vi "HEWH Check Full Credit Draw.vi"(7 "Draw_Start":dbl, 8 "error in (no error)":errorcluster, 10 "Upper Most Element":T1=enum."Lower Element", 11 "UEF Calculated Values Input in":T2 {"Data Indexes"."15 sec after Draw Index" format="%#.2f"; "Data Indexes"."15 sec after Draw Timestamp" format="%#.2f"; "Data Indexes"."Test Start Timestamp" format="%.2f"; "Data Indexes"."Test End Timestamp" format="%.2f"; "Data Indexes"."T0 Timestamp" format="%.2f"; "Data Indexes"."Tsf Timestamp" format="%.2f"; "Data Indexes"."Tsu0 Timestamp" format="%.2f"; "Data Indexes"."Tmax1 Timestamp" format="%.2f"; "Data Indexes"."Draw Index Timestamp" format="%#.2f"; "Data Indexes"."Non-Draw Timestamp" format="%#.2f"; "Data Indexes"."Heating Timestamp" format="%#.2f"; "Data Indexes"."Start Energy (BTU-Gas)" format="%.6f"; "Data Indexes"."Start Watt Hours" format="%.6f"; "Static Data"."V - Volume of Wh (True)" format="%.5f"; "Static Data"."T-Ambinet Nominal (°F)" format="%.5f"; "Static Data"."T-Inlet Setpoint (°F)" format="%.5f"; "Static Data"."T-Wh Setpoint (°F)" format="%.5f"; "Sampled Data"."Qe (Wh)" format="%.5f"; "Sampled Data"."Tau stby2 (hr)" format="%.5f"; "Sampled Data"."Tastby2 (°F)" format="%.5f"; "Sampled Data"."Qf (BTU)" format="%.5f"; "Sampled Data"."Qe (BTU)" format="%.5f"; "Sampled Data"."Tmax1 (°F)" format="%.5f"; "Sampled Data"."T0 (°F)" format="%.5f"; "Sampled Data"."Qr (BTU)" format="%.5f"; "Sampled Data"."T 24(°F)" format="%.5f"; "Sampled Data"."T astby(°F)" format="%.5f"; "Sampled Data"."T tstby(°F)" format="%.5f"; "Sampled Data"."T su0(°F)" format="%.5f"; "Sampled Data"."T suf(°F)" format="%.5f"; "Sampled Data"."Tau stby_1 (hr)" format="%.5f"; "Sampled Data"."Qsuf (BTU)" format="%.5f"; "Sampled Data"."Qsu0 (BTU)" format="%.5f"; "Calculated Values"."Draw Bonus Volume (gal)" format="%.6f"; "Calculated Values"."Adjustment Factor" format="%.6f"; "Calculated Values"."T*avg_del(n-1)" format="%.6f"; "Calculated Values"."T*min(n-1)" format="%.6f"; "Calculated Values"."T*avg_del(n)" format="%.6f"; "Calculated Values"."Vn" format="%.6f"; "Calculated Values"."Qdm (BTU)" format="%.6f"; "Calculated Values"."QHWD (BTU)" format="%.6f"; "Calculated Values"."QHW (BTU)" format="%.6f"; "Calculated Values"."UEF" format="%.6f"; "Calculated Values"."QHW67 (BTU)" format="%.6f"; "Calculated Values"."Qda (BTU)" format="%.6f"; "Calculated Values"."Qd (BTU)" format="%.6f"; "Calculated Values"."Q (BTU)" format="%.6f"; "Calculated Values"."UA (BTU/(hr*F))" format="%.6f"; "Calculated Values"."Qhr (BTU/hr)" format="%.6f"; "Calculated Values"."Qstby (BTU)" format="%.6f"; "Calculated Values"."nu_r" format="%.6f"; "Calculated Values"."CpUEF (BTU/(lb*F))" format="%.6f"; "Calculated Values"."rho_nu (lb/gal)" format="%.6f"; "Calculated Values"."V1- Vol (Gal)" format="%.6f"; "Calculated Values"."M cluster mass removed (lb)" format="%.6f"; "Calculated Values"."Cp theoretical (BTU/(lbm °F))" format="%.6f"; "Calculated Values"."Tin1 - Mean Inlet 1st Cluster (°F)" format="%.6f"; "Calculated Values"."Tdel1-Mean Outlet 1st Cluster(°F)" format="%.6f"; "Calculated Values"."Cp 24 (BTU/(lb*F))" format="%.6f"; "Calculated Values"."Cp standby (BTU/(lb*F))" format="%.6f"; "Calculated Values"."Cp2 (BTU/(lb*F))" format="%.6f"; "Calculated Values"."Cp1 (BTU/(lb*F))" format="%.6f"; "Calculated Values"."rho 24 (lb/gal)" format="%.6f"; "Calculated Values"."rho standby (lb/gal)" format="%.6f"; "Calculated Values"."rho 2 (lb/gal)" format="%.6f"; "Calculated Values"."Density of cold water All (lbm/gal)" format="%#.3g"; "Calculated Values"."CpHW (BTU/(lbm °F))" format="%#.3g"; "Calculated Values"."Density of hot water All (lbm/gal)" format="%#.3g"; "Calculated Values"."Mass of water All (lbm)" format="%#.3f"}) -> (0 "error out":errorcluster, 2 "Flow Type":T4, 3 "UEF Calculated Values Output":T2 {"Data Indexes"."15 sec after Draw Index" format="%#.2f"; "Data Indexes"."15 sec after Draw Timestamp" format="%#.2f"; "Data Indexes"."Test Start Timestamp" format="%.2f"; "Data Indexes"."Test End Timestamp" format="%.2f"; "Data Indexes"."T0 Timestamp" format="%.2f"; "Data Indexes"."Tsf Timestamp" format="%.2f"; "Data Indexes"."Tsu0 Timestamp" format="%.2f"; "Data Indexes"."Tmax1 Timestamp" format="%.2f"; "Data Indexes"."Draw Index Timestamp" format="%#.2f"; "Data Indexes"."Non-Draw Timestamp" format="%#.2f"; "Data Indexes"."Heating Timestamp" format="%#.2f"; "Data Indexes"."Start Energy (BTU-Gas)" format="%.6f"; "Data Indexes"."Start Watt Hours" format="%.6f"; "Static Data"."V - Volume of Wh (True)" format="%.5f"; "Static Data"."T-Ambinet Nominal (°F)" format="%.5f"; "Static Data"."T-Inlet Setpoint (°F)" format="%.5f"; "Static Data"."T-Wh Setpoint (°F)" format="%.5f"; "Sampled Data"."Qe (Wh)" format="%.5f"; "Sampled Data"."Tau stby2 (hr)" format="%.5f"; "Sampled Data"."Tastby2 (°F)" format="%.5f"; "Sampled Data"."Qf (BTU)" format="%.5f"; "Sampled Data"."Qe (BTU)" format="%.5f"; "Sampled Data"."Tmax1 (°F)" format="%.5f"; "Sampled Data"."T0 (°F)" format="%.5f"; "Sampled Data"."Qr (BTU)" format="%.5f"; "Sampled Data"."T 24(°F)" format="%.5f"; "Sampled Data"."T astby(°F)" format="%.5f"; "Sampled Data"."T tstby(°F)" format="%.5f"; "Sampled Data"."T su0(°F)" format="%.5f"; "Sampled Data"."T suf(°F)" format="%.5f"; "Sampled Data"."Tau stby_1 (hr)" format="%.5f"; "Sampled Data"."Qsuf (BTU)" format="%.5f"; "Sampled Data"."Qsu0 (BTU)" format="%.5f"; "Calculated Values"."Draw Bonus Volume (gal)" format="%.6f"; "Calculated Values"."Adjustment Factor" format="%.6f"; "Calculated Values"."T*avg_del(n-1)" format="%.6f"; "Calculated Values"."T*min(n-1)" format="%.6f"; "Calculated Values"."T*avg_del(n)" format="%.6f"; "Calculated Values"."Vn" format="%.6f"; "Calculated Values"."Qdm (BTU)" format="%.6f"; "Calculated Values"."QHWD (BTU)" format="%.6f"; "Calculated Values"."QHW (BTU)" format="%.6f"; "Calculated Values"."UEF" format="%.6f"; "Calculated Values"."QHW67 (BTU)" format="%.6f"; "Calculated Values"."Qda (BTU)" format="%.6f"; "Calculated Values"."Qd (BTU)" format="%.6f"; "Calculated Values"."Q (BTU)" format="%.6f"; "Calculated Values"."UA (BTU/(hr*F))" format="%.6f"; "Calculated Values"."Qhr (BTU/hr)" format="%.6f"; "Calculated Values"."Qstby (BTU)" format="%.6f"; "Calculated Values"."nu_r" format="%.6f"; "Calculated Values"."CpUEF (BTU/(lb*F))" format="%.6f"; "Calculated Values"."rho_nu (lb/gal)" format="%.6f"; "Calculated Values"."V1- Vol (Gal)" format="%.6f"; "Calculated Values"."M cluster mass removed (lb)" format="%.6f"; "Calculated Values"."Cp theoretical (BTU/(lbm °F))" format="%.6f"; "Calculated Values"."Tin1 - Mean Inlet 1st Cluster (°F)" format="%.6f"; "Calculated Values"."Tdel1-Mean Outlet 1st Cluster(°F)" format="%.6f"; "Calculated Values"."Cp 24 (BTU/(lb*F))" format="%.6f"; "Calculated Values"."Cp standby (BTU/(lb*F))" format="%.6f"; "Calculated Values"."Cp2 (BTU/(lb*F))" format="%.6f"; "Calculated Values"."Cp1 (BTU/(lb*F))" format="%.6f"; "Calculated Values"."rho 24 (lb/gal)" format="%.6f"; "Calculated Values"."rho standby (lb/gal)" format="%.6f"; "Calculated Values"."rho 2 (lb/gal)" format="%.6f"; "Calculated Values"."Density of cold water All (lbm/gal)" format="%#.3g"; "Calculated Values"."CpHW (BTU/(lbm °F))" format="%#.3g"; "Calculated Values"."Density of hot water All (lbm/gal)" format="%#.3g"; "Calculated Values"."Mass of water All (lbm)" format="%#.3f"})   [LabVIEW 2023]
uses:
  Type Definitions/HEWH FHR Draw Type.ctl
  Type Definitions/UEF Constants.ctl
  Type Definitions/HEWH Draw Stats.ctl
  Type Definitions/FHR Bins.ctl
  Type Definitions/HEWH Meter Type.ctl
  Type Definitions/Upper Most Element.ctl
panel:
  out "Time Heating Turned Off":dbl
  # "FHR"
  # "FHR"
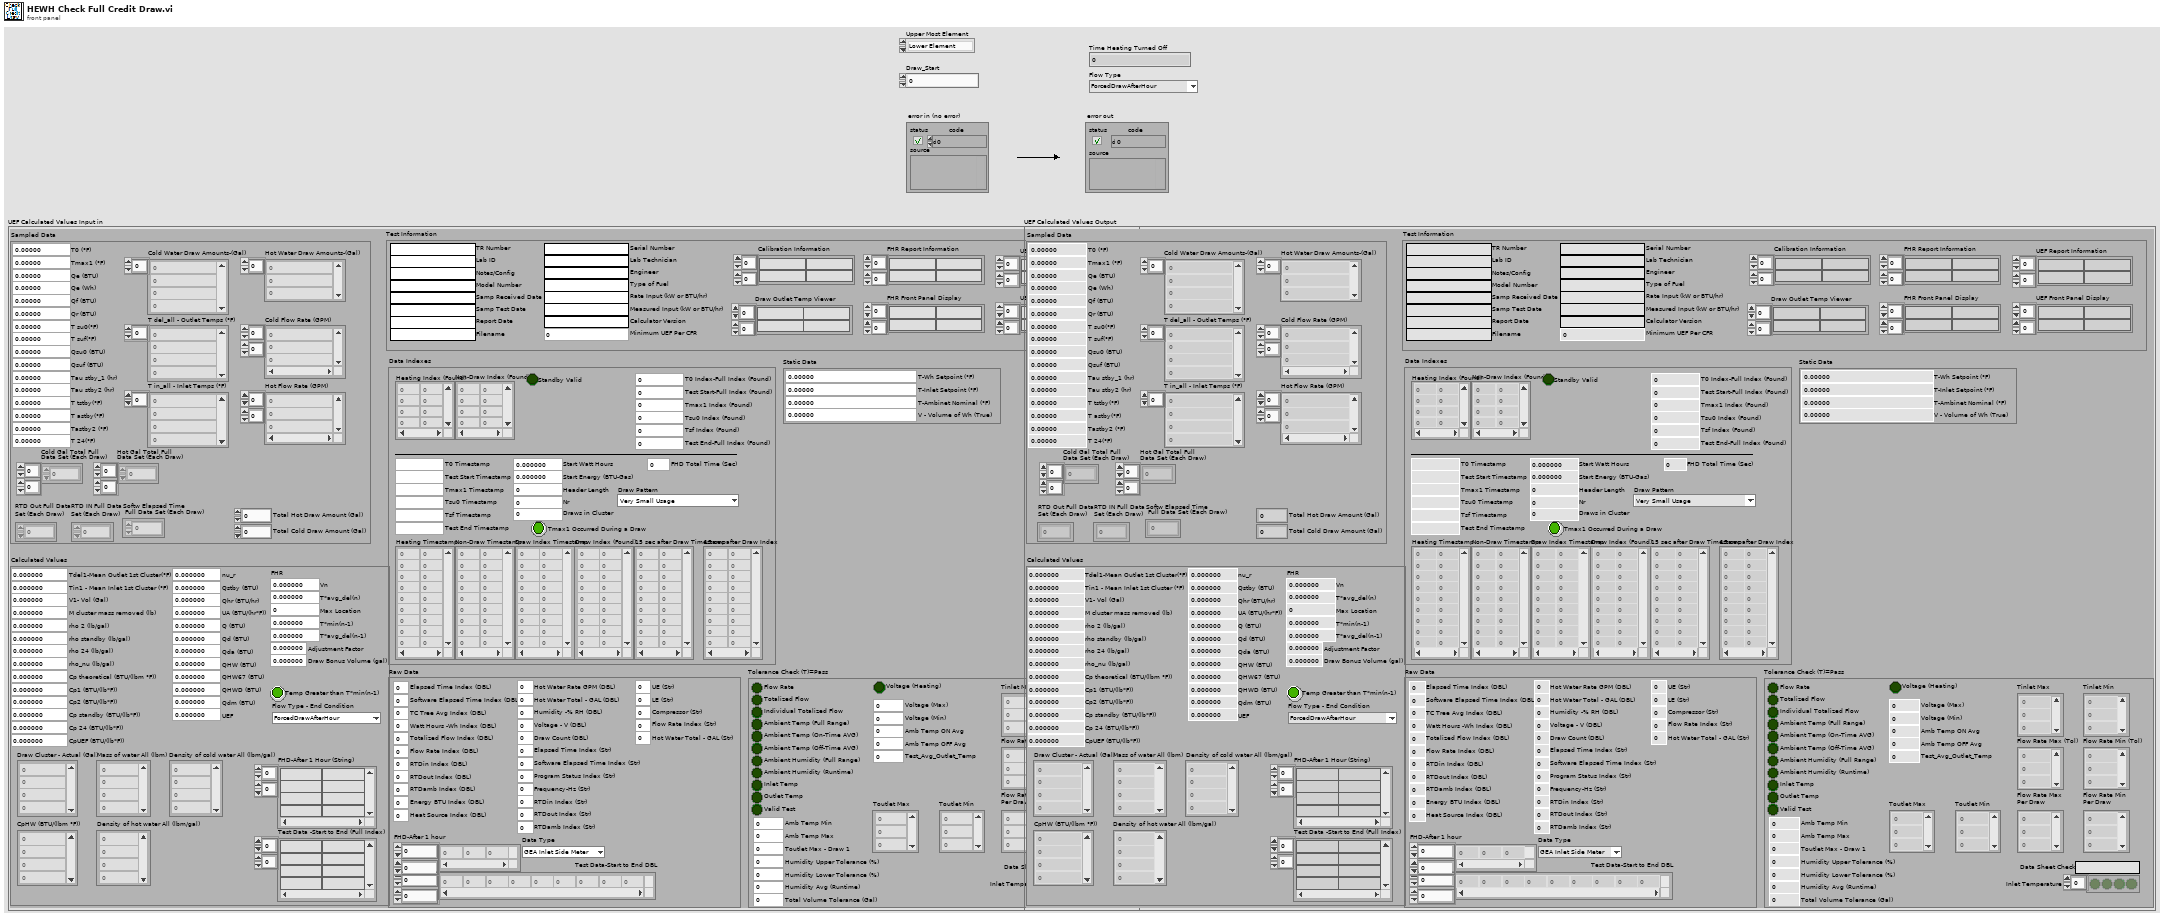
[diagram p1: front panel]
types:
  T1 = typedef "Upper Most Element.ctl" = enum16{"Compressor", "Lower Element", "Upper Element"}
  T2 = typedef "UEF Constants.ctl" = cluster{"Calculated Values":T3, "Sampled Data":cluster{"Cold Water Draw Amounts-(Gal)":dbl[], "T del_all - Outlet Temps (°F)":dbl[], "T in_all - Inlet Temps (°F)":dbl[], "Qsu0 (BTU)":dbl, "Qsuf (BTU)":dbl, "Tau stby_1 (hr)":dbl, "T suf(°F)":dbl, "T su0(°F)":dbl, "T tstby(°F)":dbl, "T astby(°F)":dbl, "T 24(°F)":dbl, "Qr (BTU)":dbl, "T0 (°F)":dbl, "Tmax1 (°F)":dbl, "Qe (BTU)":dbl, "Qf (BTU)":dbl, "Tastby2 (°F)":dbl, "RTD Out Full Data\nSet (Each Draw)":dbl[][], "RTD IN Full Data\nSet (Each Draw)":dbl[][], "Tau stby2 (hr)":dbl, "Hot Water Draw Amounts-(Gal)":dbl[], "Cold Flow Rate (GPM)":dbl[][], "Hot Flow Rate (GPM)":dbl[][], "Softw Elapsed Time\n Full Data Set (Each Draw)":dbl[][], "Cold Gal Total Full\nData Set (Each Draw)":dbl[][], "Total Hot Draw Amount (Gal) ":dbl, "Total Cold Draw Amount (Gal)":dbl, "Qe (Wh)":dbl, "Hot Gal Total Full\nData Set (Each Draw)":dbl[][]}, "Static Data":cluster{"T-Wh Setpoint (°F)":dbl, "T-Inlet Setpoint (°F)":dbl, "T-Ambinet Nominal (°F)":dbl, "V - Volume of Wh (True)":dbl}, "Data Indexes":cluster{"Test Start-Full Index (Found)":i32, "Header Length":i32, "Draw Index (Found)":i32[][], "Nr":i32, "Start Watt Hours":dbl, "Tsu0 Index (Found)":i32, "Tsf Index (Found)":i32, "Start Energy (BTU-Gas)":dbl, "Draws in Cluster":i32, "T0 Index-Full Index (Found)":i32, "Non-Draw Index (Found)":i32[][], "Tmax1 Index (Found)":i32, "Test End-Full Index (Found)":i32, "Heating Index (Found)":i32[][], "Heating Timestamp":dbl[][], "Non-Draw Timestamp":dbl[][], "Draw Index Timestamp":dbl[][], "Tmax1 Timestamp":dbl, "Tsu0 Timestamp":dbl, "Tsf Timestamp":dbl, "T0 Timestamp":dbl, "Test End Timestamp":dbl, "Test Start Timestamp":dbl, "15 sec after Draw Timestamp":dbl[][], "15 sec after Draw Index":dbl[][], "Tmax1 Occurred During a Draw":bool, "FHD Total Time (Sec)":dbl, "Draw Pattern":T5, "Standby Valid":bool}, "Raw Data":cluster{"Elapsed Time Index (DBL)":i32, "Software Elapsed Time Index (DBL)":i32, "TC Tree Avg Index (DBL)":i32, "Watt Hours -Wh Index (DBL)":i32, "Energy BTU Index (DBL)":i32, "Totalized Flow Index (DBL)":i32, "Flow Rate Index (DBL)":i32, "Program Status Index (Str)":i32, "RTDin Index (DBL)":i32, "RTDout Index (DBL)":i32, "RTDamb Index (DBL)":i32, "Test Data-Start to End DBL":dbl[][], "Data Type":T6, "Heat Source Index (DBL)":i32, "Hot Water Rate GPM (DBL)":i32, "Hot Water Total - GAL (DBL)":i32, "FHD-After 1 hour":dbl[][], "Humidity -% RH (DBL)":i32, "Voltage - V (DBL)":i32, "Draw Count (DBL)":i32, "Elapsed Time Index (Str)":i32, "Software Elapsed Time Index (Str)":i32, "Frequency-Hz (Str)":i32, "RTDin Index (Str)":i32, "RTDout Index (Str)":i32, "RTDamb Index (Str)":i32, "UE (Str)":i32, "LE (Str)":i32, "Compressor (Str)":i32, "Flow Rate Index (Str)":i32, "Hot Water Total - GAL (Str)":i32}, "Tolerance Check (T)=Pass":cluster{"Flow Rate":bool, "Totalized Flow":bool, "Ambient Temp (Full Range)":bool, "Ambient Humidity (Full Range)":bool, "Inlet Temp":bool, "Outlet Temp":bool, "Valid Test":bool, "Individual Totalized Flow":bool, "Data Sheet Check":string, "Inlet Temperature":bool[], "Tinlet Max":dbl[], "Tinlet Min":dbl[], "Flow Rate Max (Tol)":dbl[], "Flow Rate Min (Tol)":dbl[], "Amb Temp Max":dbl, "Amb Temp Min":dbl, "Toutlet Max - Draw 1":dbl, "Humidity Upper Tolerance (%)":dbl, "Total Volume Tolerance (Gal)":dbl, "Humidity Lower Tolerance (%)":dbl, "Flow Rate Max\nPer Draw":dbl[], "Flow Rate Min\nPer Draw":dbl[], "Ambient Humidity (Runtime)":bool, "Humidity Avg (Runtime)":dbl, "Ambient Temp (On-Time AVG)":bool, "Ambient Temp (Off-Time AVG)":bool, "Amb Temp OFF Avg":dbl, "Amb Temp ON Avg":dbl, "Voltage (Heating)":bool, "Voltage (Min)":dbl, "Voltage (Max)":dbl, "Toutlet Max":dbl[], "Toutlet Min":dbl[], "Test_Avg_Outlet_Temp":dbl}, "Test Information":cluster{"TR Number":string, "Lab ID":string, "Notes/Config":string, "Model Number":string, "Serial Number":string, "Lab Technician":string, "Engineer":string, "Type of Fuel":string, "Samp Received Date":string, "Samp Test Date":string, "Report Date":string, "Rate Input (kW or BTU/hr)":string, "Measured Input (kW or BTU/hr)":string, "Filename":string, "Calibration Information":string[][], "Calculator Version":string, "Minimum UEF Per CFR":dbl, "UEF Report Information":string[][], "FHR Report Information":string[][], "FHR Front Panel Display":string[][], "UEF Front Panel Display":string[][], "Draw Outlet Temp Viewer":string[][]}}
  T3 = typedef "HEWH Draw Stats.ctl" = cluster{"Draw Cluster - Actual (Gal)":dbl[], "Mass of water All (lbm)":dbl[], "Density of hot water All (lbm/gal)":dbl[], "CpHW (BTU/(lbm °F))":dbl[], "rho 2 (lb/gal)":dbl, "rho standby (lb/gal)":dbl, "rho 24 (lb/gal)":dbl, "Cp1 (BTU/(lb*F))":dbl, "Cp2 (BTU/(lb*F))":dbl, "Cp standby (BTU/(lb*F))":dbl, "Cp 24 (BTU/(lb*F))":dbl, "nu_r":dbl, "Qstby (BTU)":dbl, "Qhr (BTU/hr)":dbl, "UA (BTU/(hr*F))":dbl, "Q (BTU)":dbl, "Qd (BTU)":dbl, "Qda (BTU)":dbl, "QHW67 (BTU)":dbl, "UEF":dbl, "Tdel1-Mean Outlet 1st Cluster(°F)":dbl, "Tin1 - Mean Inlet 1st Cluster (°F)":dbl, "Cp theoretical (BTU/(lbm °F))":dbl, "M cluster mass removed (lb)":dbl, "V1- Vol (Gal)":dbl, "Test Data -Start to End (Full Index)":string[][], "rho_nu (lb/gal)":dbl, "Density of cold water All (lbm/gal)":dbl[], "CpUEF (BTU/(lb*F))":dbl, "QHW (BTU)":dbl, "QHWD (BTU)":dbl, "Qdm (BTU)":dbl, "FHD-After 1 Hour (String)":string[][], "Vn":dbl, "T*avg_del(n)":dbl, "Max Location":i32, "T*min(n-1)":dbl, "T*avg_del(n-1)":dbl, "Temp Greater than T*min(n-1)":bool, "Adjustment Factor":dbl, "Draw Bonus Volume (gal)":dbl, "Flow Type - End Condition":T4}
  T4 = typedef "HEWH FHR Draw Type.ctl" = enum16{"ForcedDrawAfterHour", "HeatingCutoffBeforeHour"}
  T5 = typedef "FHR Bins.ctl" = enum16{"Very Small Usage", "Low Usage", "Medium Usage", "High Usage", "Undefined"}
  T6 = typedef "HEWH Meter Type.ctl" = enum16{"GEA Inlet Side Meter", "GEA Outlet Side Meter", "CSA Inlet Side Meter"}
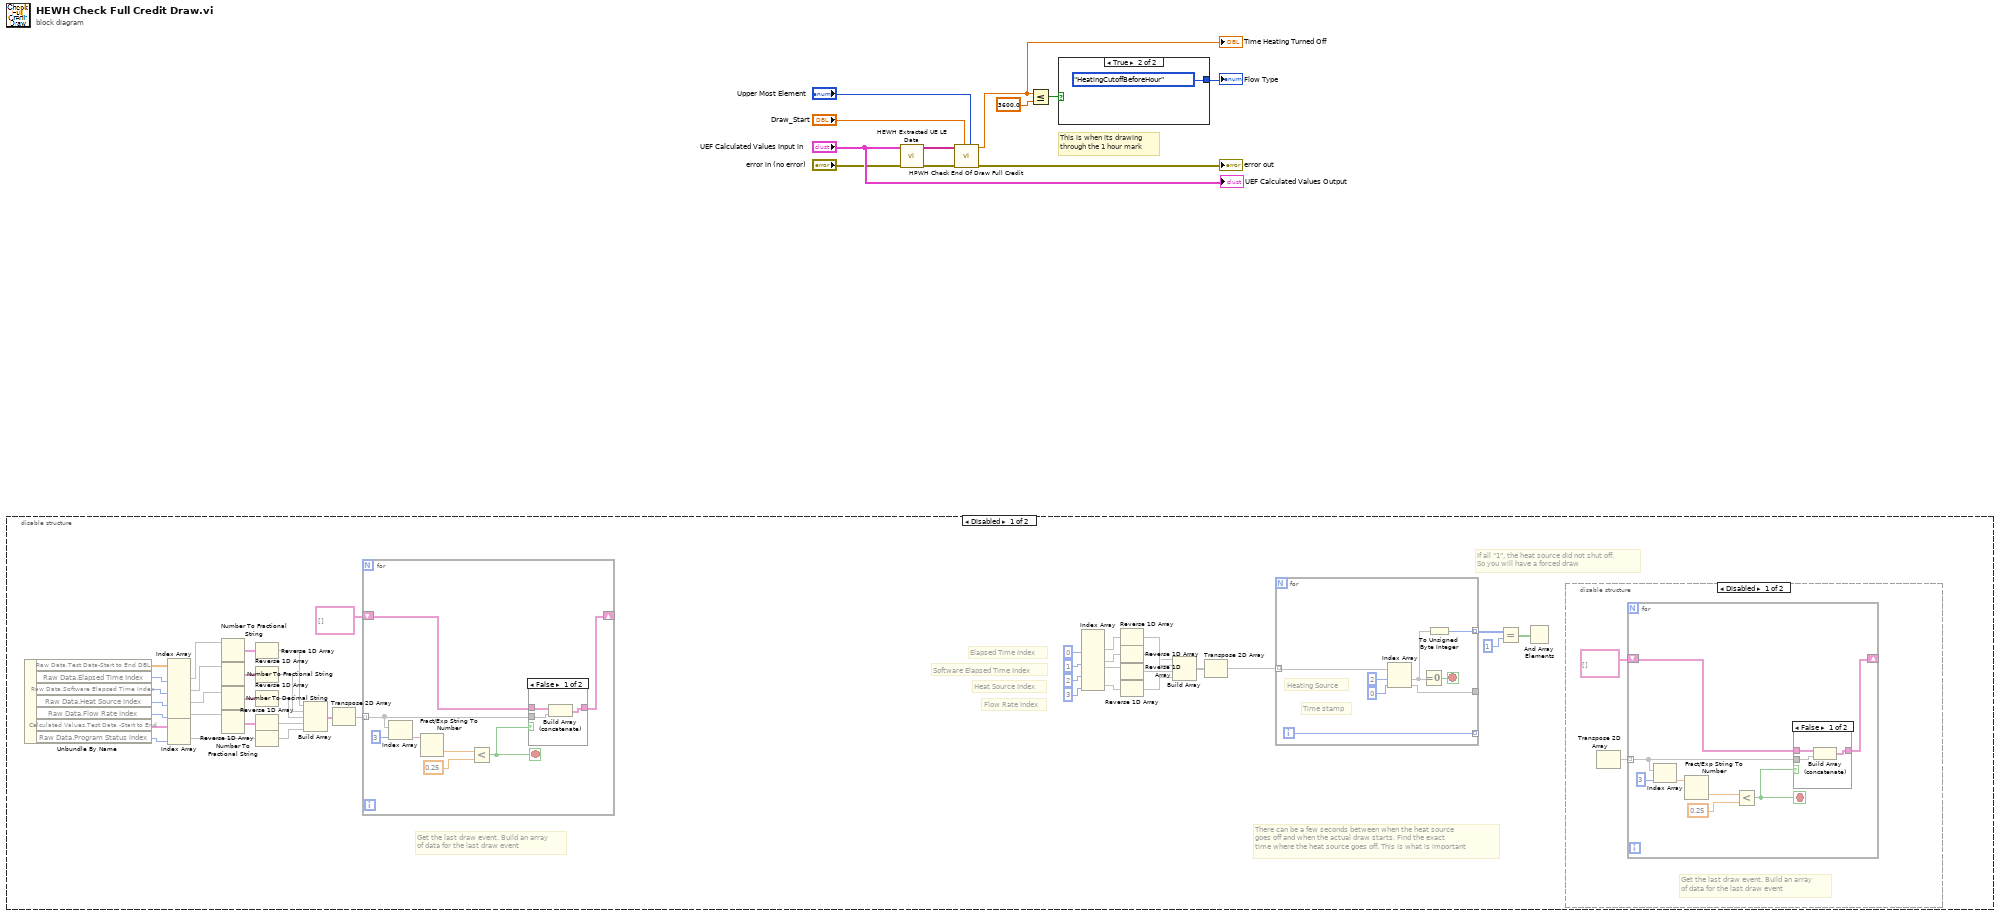
[diagram p0: block diagram]
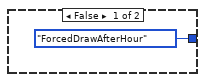
[diagram p2: hidden frame]
diagram:
  # "This is when its drawing\nthrough the 1 hour mark"
  n1 = disable-structure shown="Disabled" {
    frame Disabled {
      # "Get the last draw event. Build an array\nof data for the last draw event"
      # "If all \"1\", the heat source did not shut off.\nSo you will have a forced draw"
      # "Flow Rate Index"
      # "Heat Source Index"
      # "Software Elapsed Time Index"
      # "Elapsed Time Index"
      # "There can be a few seconds between when the heat source\ngoes off and when the actual draw starts. Find the exact\ntime where the heat source goes off. This is what is important"
      n2 = Unbundle By Name() -> ("Raw Data.Test Data-Start to End DBL"=w17:dbl[][], "Raw Data.Elapsed Time Index"=w16:i32, "Raw Data.Software Elapsed Time Index"=w15:i32, "Raw Data.Heat Source Index"=w14:i32, "Raw Data.Flow Rate Index"=w13:i32, "Calculated Values.Test Data -Start to End"=w24:string[][], "Raw Data.Program Status Index"=w25:i32)  [unwired: 1 in]
      n3 = Index Array(array=w17, index (col) #1=w16, index (col) #2=w15, index (col) #3=w14, index (col) #4=w13) -> (element #1=w27:dbl[], element #2=w29:dbl[], element #3=w31:dbl[], element #4=w33:dbl[])  [unwired: 4 in]
      n4 = Index Array(array=w24, index (col)=w25) -> (element=w26:string[])  [unwired: 1 in]
      n5 = Number To Fractional String(number=w27) -> (F-format string=w28:string[])  [unwired: 3 in]
      n6 = Number To Fractional String(number=w29) -> (F-format string=w30:string[])  [unwired: 3 in]
      n7 = Number To Decimal String(number=w31) -> (decimal integer string=w32:string[])  [unwired: 1 in]
      n8 = Number To Fractional String(number=w33) -> (F-format string=w34:string[])  [unwired: 3 in]
      n9 = Reverse 1D Array(array=w28) -> (reversed array=w21:string[])
      n10 = Reverse 1D Array(array=w30) -> (reversed array=w20:string[])
      n11 = Reverse 1D Array(array=w32) -> (reversed array=w19:string[])
      n12 = Reverse 1D Array(array=w34) -> (reversed array=w18:string[])
      n13 = Reverse 1D Array(array=w26) -> (reversed array=w23:string[])
      n14 = Build Array(w21, w20, w19, w18, w23) -> (w22:string[][])
      n15 = Transpose 2D Array(2D array=w22) -> (transposed array=w35:string[][])
      n16 = for {
        tunnel: w35 -> [w70] mode=indexing
        shift-right: [w71] -> _
        shift-left: string[][] [] -> [w72]
        stop <- w73 stop-if-true
        n17 = Index Array(array=w70, index=3) -> (element=w69:string)
        n18 = Fract/Exp String To Number(string=w69) -> (number=w67:dbl)  [unwired: 3 in, 1 out]
        n19 = Less?(x=w67, y=0.25) -> (x < y?=w73:bool)
        n20 = case shown="False" w73 {
          tunnel: [w76 w78] -> w71
          tunnel: w72 -> [w77 w78]
          tunnel: w70 -> [w75 _]
          frame False {
            n21 = Build Array (concatenate)(w77, w75) -> (w76:string[][])
          }
          frame True {
          }
        }
      }
      n22 = Index Array(index (col) #1=0 ("disabled index (col)"), index (col) #2=1 ("index (col)"), index (col) #3=2 ("index (col)"), index (col) #4=3 ("index (col)")) -> (element #1=w44, element #2=w45, element #3=w46, element #4=w47)  [unwired: 5 in]
      n23 = Reverse 1D Array(array=w44) -> (reversed array=w49:void[])
      n24 = Reverse 1D Array(array=w45) -> (reversed array=w50:void[])
      n25 = Reverse 1D Array(array=w46) -> (reversed array=w51:void[])
      n26 = Reverse 1D Array(array=w47) -> (reversed array=w52:void[])
      n27 = Build Array(w49, w50, w51, w52) -> (w48:void[])
      n28 = Transpose 2D Array(2D array=w48) -> (transposed array=w36:void[][])
      n29 = for {
        tunnel: w36 -> [w85] mode=indexing
        tunnel: [w82] -> _
        tunnel: [w81] -> _ mode=indexing
        tunnel: [w79] -> w39 mode=indexing
        i -> [w81]
        stop <- w84 stop-if-true
        # "Time stamp"
        # "Heating Source"
        n30 = Index Array(array=w85, index #1=2 ("index"), index #2=0 ("index")) -> (element #1=w80, element #2=w82)
        n31 = Equal To 0?(x=w80) -> (x = 0?=w84:bool)
        n32 = To Unsigned Byte Integer(number=w80) -> (unsigned 8bit integer=w79:u8)
      }
      n33 = Equal?(x=w39, y=u8 1) -> (x = y?=w37:bool[])
      n34 = And Array Elements(Boolean array=w37) -> ()  [unwired: 1 out]
      n35 = disable-structure shown="Disabled" {
        frame Disabled {
          # "Get the last draw event. Build an array\nof data for the last draw event"
          n36 = Transpose 2D Array() -> (transposed array=w53:dbl[][])  [unwired: 1 in]
          n37 = for {
            tunnel: w53 -> [w58] mode=indexing
            shift-right: [w59] -> _
            shift-left: string[][] [] -> [w60]
            stop <- w61 stop-if-true
            n38 = Index Array(array=w58, index=3) -> (element=w57:dbl)
            n39 = Fract/Exp String To Number(string=w57) -> (number=w55:dbl)  [unwired: 3 in, 1 out]
            n40 = Less?(x=w55, y=0.25) -> (x < y?=w61:bool)
            n41 = case shown="False" w61 {
              tunnel: [w64 w66] -> w59
              tunnel: w60 -> [w65 w66]
              tunnel: w58 -> [w63 _]
              frame False {
                n42 = Build Array (concatenate)(w65, w63) -> (w64:string[][])
              }
              frame True {
              }
            }
          }
        }
        frame Enabled {
        }
      }
    }
    frame Enabled {
    }
  }
  n43 = call "HEWH Extracted UE LE Data.vi"("error in (no error)"="error in (no error)", "UEF Calculated Values Input in"="UEF Calculated Values Input in") -> ("error out"=w2:errorcluster, "Extracted UE LE Data"=w10:string[][])  [unwired: 8 in]
  n44 = call "HPWH Check End Of Draw Full Credit.vi"("Upper Most Element"="Upper Most Element", "Draw_Start"="Draw_Start", "error in (no error)"=w2, "Test Start to End"=w10) -> ("error out"=→"error out":errorcluster, "Cutout Time (Seconds)"=w6:dbl)  [unwired: 6 in]
  "Time Heating Turned Off" <- w6
  n45 = Less Or Equal?(x=w6, y=3600.0) -> (x <= y?=w8:bool)
  n46 = case shown="True" w8 {
    tunnel: [HEWH_FHR_Draw_Type."ForcedDrawAfterHour" ("Flow Type") HEWH_FHR_Draw_Type."HeatingCutoffBeforeHour" ("Flow Type")] -> w9
    frame False {
    }
    frame True {
    }
  }
  "Flow Type" <- w9
  "UEF Calculated Values Output" <- "UEF Calculated Values Input in"
